vi "Wait For Plugin Command.vi"(8 "error in (no error)":errorcluster, 9 "timeout in ms (0)":i32, 11 "Plugin Interface in":refnum<class "Plugin Interface.lvclass">) -> (0 "error out":errorcluster, 2 "command":T1={"Command"=enum."Rx", "Parameters"={"arg1"=0, "arg2"=0}}, 3 "Plugin Interface out":refnum<class "Plugin Interface.lvclass">, 4 "# elements":u32)   [LabVIEW 2017, in "DSF Core.lvlib" / "Plugin Interface.lvclass"]
uses:
  Plugin Interface.lvclass
  C:/Git/DSF/Data Sharing Framework/Source/Core/Engine/Classes/Interfaces/Interface/Interface.lvclass
  Command Data.ctl
  Command.ctl
  Command Parameters.ctl
  Interface/Interface.lvclass/Interface.ctl
  Interface/Read RT FIFO.vi
  Dispatcher/Command Timeout.vi
  Interface/Interface.lvclass
  DSF Core.lvlib
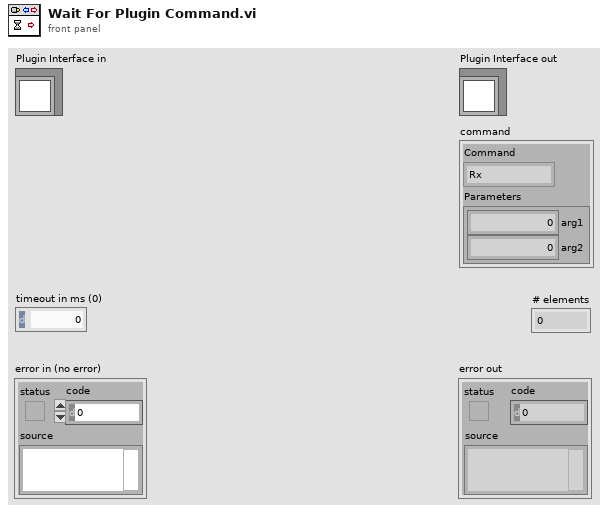
[diagram p1: front panel]
types:
  T1 = typedef "DSF Core.lvlib/Plugin Interface.lvclass/Command Data.ctl" = cluster{"Command":T2, "Parameters":T3}
  T2 = typedef "DSF Core.lvlib/Plugin Interface.lvclass/Command.ctl" = enum8{"Set Inline Buffer", "Rx", "Tx", "Shutdown"}
  T3 = typedef "DSF Core.lvlib/Plugin Interface.lvclass/Command Parameters.ctl" = cluster{"arg1":u64, "arg2":u64}
  T4 = typedef "DSF Core.lvlib/Interface.lvclass/RT FIFO Data.ctl" = cluster{"Command":u8, "Parameters":T5}
  T5 = typedef "DSF Core.lvlib/Interface.lvclass/RT FIFO Parameters.ctl" = cluster{"arg1":u64, "arg2":u64}
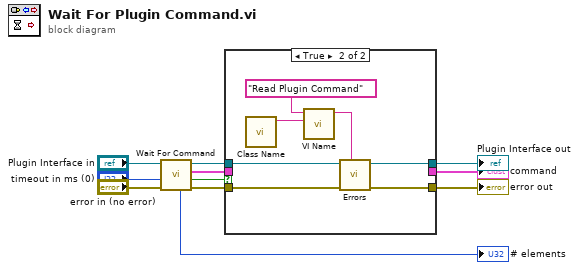
[diagram p0: block diagram]
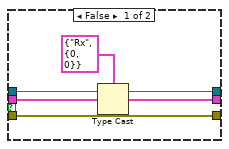
[diagram p2: hidden frame]
diagram:
  n1 = call "Wait For Command.vi"("error in (no error)"="error in (no error)", "timeout in ms (0)"="timeout in ms (0)", "Interface in"="Plugin Interface in") -> ("error out"=w7:errorcluster, "timed out?"=w5:bool, "command"=w6:T4, "Interface out"=w8:refnum<class "Plugin Interface.lvclass">, "# elements"=→"# elements":u32)  [unwired: 4 in]
  n2 = case shown="True" w5 {
    tunnel: [w15 _] -> w2
    tunnel: w6 -> [w14 _]
    tunnel: w8 -> [w16 w17]
    tunnel: [w16 w22] -> w4
    tunnel: w7 -> [w13 w23]
    tunnel: [w13 w21] -> w3
    frame False {
      n3 = Type Cast(type=T1 {"Command"=enum."Rx", "Parameters"={"arg1"=0, "arg2"=0}} ("Plugin Command"), x=w14) -> (*(type *) &x=w15:T1)
    }
    frame True {
      n4 = call "Class Name.vi"() -> ("class name"=w19:string)  [unwired: 11 in]
      n5 = call "VI Name.vi"("class name (\"\")"=w19, "vi name"="Read Plugin Command" ("error source vi name")) -> ("full VI name"=w18:string)  [unwired: 9 in]
      n6 = call-poly "Errors.vi"("error source vi name"=w18, "error in (no error)"=w23, "Interface in"=w17) -> ("error out"=w21:errorcluster, "Interface out"=w22:refnum<class "Plugin Interface.lvclass">)  [unwired: 7 in]
    }
  }
  "error out" <- w3
  "Plugin Interface out" <- w4
  "command" <- w2
